vi "S_Curve.vi"(8 "error in (no error)":errorcluster caption="entrée d'erreur (pas d'erreur)", 11 "make_s_curve":T2={"n_samples"=100, "noise"=0.0, "random_state"=-1, "Returns"="X"} {"random_state" min=-1; "n_samples" min=1}) -> (0 "error out":errorcluster, 3 "Data":T1)   [LabVIEW 2020]
doc: "Generate an S curve dataset.\n\n\nParameters :\n\n- n_samples : int, optional (default=100)\nThe number of sample points on the S curve.\n\n- noise : float, optional (default=0.0)\nThe standard deviation of the gaussian noise.\n\n- random_state : int, RandomState instance, default=None=-1\nDetermines random number generation for dataset creation. Pass an int for reproducible output across multiple function calls. See Glossary.\n\nReturns :\n\n- X : array of shape [n_samples, 3]\nThe points.\n\n- t : array of shape [n_samples]\nThe univariate position of the sample according to the main dimension of the points in the manifold."
uses:
  S_Curve.lvclass
panel:
  out "S_Curve.lvclass":refnum<class "S_Curve.lvclass">
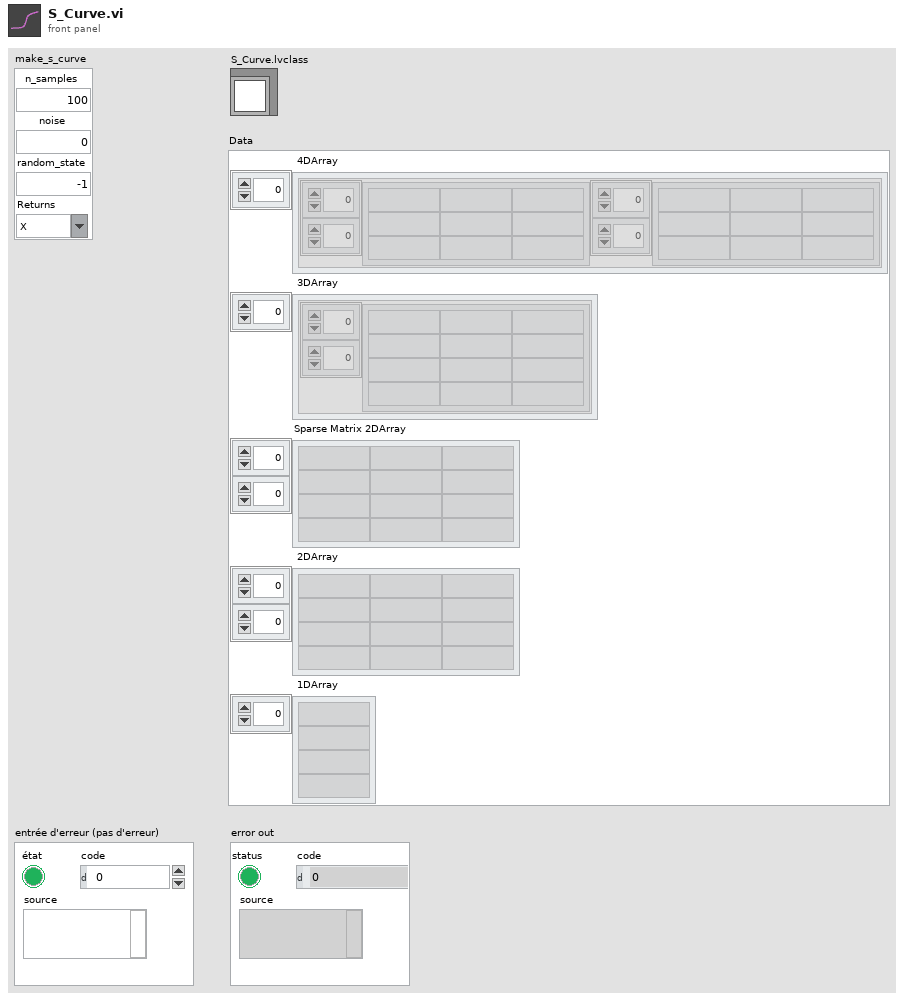
[diagram p1: front panel]
types:
  T1 = cluster{" 4DArray":cluster{"1":string[][], "2":string[][]}[], " 3DArray":cluster{"Tableau":string[][]}[], "Sparse Matrix 2DArray":string[][], " 2DArray":string[][], " 1DArray":string[]}
  T2 = cluster{"n_samples":u32, "noise":dbl, "random_state":i32, "Returns":string}
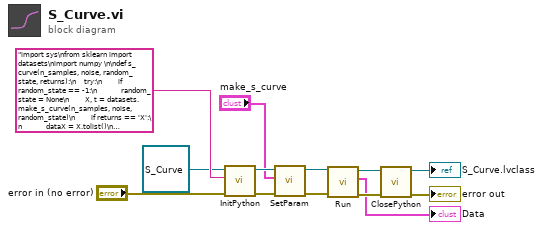
[diagram p0: block diagram]
diagram:
  n1 = call-dynamic "InitPython.vi"("error in (no error)"="error in (no error)", "Python Instruction"="import sys\nfrom sklearn import datasets\nimport numpy \n\ndef s_curve(n_samples, noise, random_state, returns):\n    try:\n        if random_state == -1:\n            random_state = None\n        X, t = datasets.make_s_curve(n_samples, noise, random_state)\n        if returns == 'X':\n            dataX = X.tolist()\n            return str(dataX)\n        else: \n            data_t = t.tolist()\n            return str(data_t)\n    except:\n        erreur = sys.exc_info()\n        typerr = u\"%s\" % (erreur[0])\n        typerr = typerr[typerr.find(\"'\")+1:typerr.rfind(\"'\")]\n        msgerr = u\"%s\" % (erreur[1])\n        message = str('/!\\\\ {0} : {1}'. format(typerr,msgerr))\n        return message", "Scikit-learn en entrée"=refnum<class "S_Curve.lvclass"> refnum ("S_Curve.lvclass")) -> ("error out"=w7:errorcluster, "Scikit-learn en sortie"=w10:refnum<class "S_Curve.lvclass">)  [unwired: 7 in]
  n2 = call-dynamic "SetParam.vi"("error in (no error)"=w7, "make_s_curve"="make_s_curve", "S_Curve.lvclass"=w10) -> ("error out"=w6:errorcluster, "S_Curve.lvclass"=w9:refnum<class "S_Curve.lvclass">)  [unwired: 7 in]
  n3 = call-dynamic "Run.vi"("error in (no error)"=w6, "S_Curve.lvclass"=w9) -> ("error out"=w5:errorcluster, "Data"=→"Data":T1, "S_Curve.lvclass"=w8:refnum<class "S_Curve.lvclass">)  [unwired: 7 in]
  n4 = call-dynamic "ClosePython.vi"("error in (no error)"=w5, "Scikit-learn en entrée"=w8) -> ("error out"=→"error out":errorcluster, "Scikit-learn en sortie"=→"S_Curve.lvclass":refnum<class "S_Curve.lvclass">)  [unwired: 8 in]
